vi "GetMsgData.vi"(8 "error in (no error)":errorcluster, 11 "Exit in":refnum<class "Exit.lvclass">) -> (0 "error out":errorcluster, 2 "MsgData":variant, 3 "Exit out":refnum<class "Exit.lvclass">)   [LabVIEW 2020, in "UpstreamMsg.lvlib" / "Exit.lvclass"]
doc: "This is used in the scripting to create the go, it provides the datatype"
uses:
  Exit.lvclass
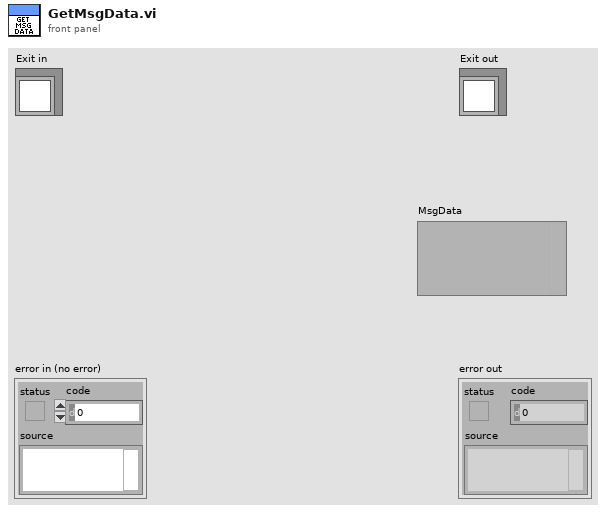
[diagram p1: front panel]
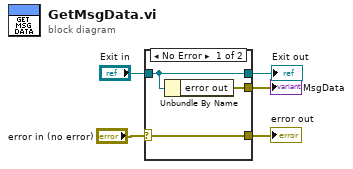
[diagram p0: block diagram]
diagram:
  n1 = case shown="No Error" "error in (no error)" {
    selector: "error in (no error)" -> [w8 w10]
    tunnel: [w8 w10] -> w5
    tunnel: [w7 w9] -> w3
    tunnel: "Exit in" -> [w7 w9]
    tunnel: [w6 _] -> w4
    frame No Error {
      n2 = Unbundle By Name(w7) -> ("error out"=w6:errorcluster)
    }
    frame Error {
    }
  }
  "error out" <- w5
  "Exit out" <- w3
  "MsgData" <- w4
